vi "GPIB Send Receive.vi"(1 "RDY max wait, ms":u32=500, 4 "RDY when up":bool=TRUE, 5 "Data ready bit (-1 - ignore)":i32=-1, 6 "Read terminator":i16, 7 "Delay, ms":u32, 8 "error in (no error)":errorcluster, 9 "Receive count":i32=256, 10 "data string in":string, 11 "GPIB Adress":i16) -> (0 "error out":errorcluster, 2 "data string out":string, 3 "GPIB Adress out":i16)   [LabVIEW 2019]
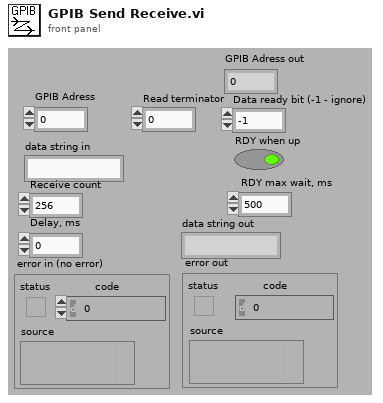
[diagram p1: front panel]
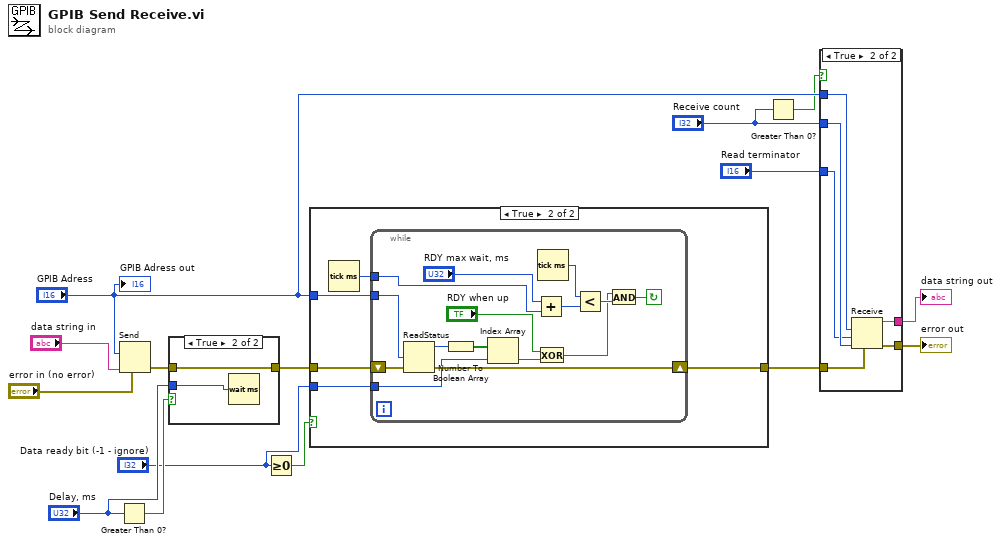
[diagram p0: block diagram]
diagram:
  n1 = Greater Than 0?(x="Delay, ms") -> (x > 0?=w11:bool)
  n2 = Send(2:"GPIB Adress", 4:"error in (no error)", 5:"data string in") -> (8:w10:errorcluster)  [unwired: 4 out]
  n3 = case shown="True" w11 {
    tunnel: w10 -> [w16 w17]
    tunnel: [w16 w17] -> w5
    tunnel: "Delay, ms" -> [_ w18]
    frame False {
    }
    frame True {
      n4 = Wait (ms)(milliseconds to wait=w18) -> ()  [unwired: 1 out]
    }
  }
  n5 = Greater Or Equal To 0?(x="Data ready bit (-1 - ignore)") -> (x >= 0?=w7:bool)
  n6 = case shown="True" w7 {
    tunnel: "GPIB Adress" -> [_ w23]
    tunnel: w5 -> [w19 w22]
    tunnel: "Data ready bit (-1 - ignore)" -> [_ w21]
    tunnel: [w19 w20] -> w3
    frame False {
    }
    frame True {
      n7 = Tick Count (ms)() -> (millisecond timer value=w24:u32)
      n8 = while {
        tunnel: w23 -> [w38]
        shift-right: [w37] -> w20
        shift-left: w22 -> [w39]
        tunnel: w24 -> [w32]
        tunnel: w21 -> [w28]
        stop <- w36 continue-if-true
        n9 = ReadStatus(3:w39, 4:w38) -> (0:w37:errorcluster, 2:w34:i16)  [unwired: 2 out]
        n10 = Number To Boolean Array(number=w34) -> (Boolean array=w30:bool[])
        n11 = Index Array(array=w30, index=w28) -> (element=w27:bool)
        n12 = Add(x="RDY max wait, ms", y=w32) -> (x+y=w33:u32)
        n13 = Exclusive Or(1:w27, 2:"RDY when up") -> (0:w26:bool)
        n14 = Tick Count (ms)() -> (millisecond timer value=w31:u32)
        n15 = Less?(x=w31, y=w33) -> (x < y?=w35:bool)
        n16 = And(x=w26, y=w35) -> (x .and. y?=w36:bool)
      }
    }
  }
  n17 = Greater Than 0?(x="Receive count") -> (x > 0?=w1:bool)
  n18 = case shown="True" w1 {
    tunnel: [w40 w46] -> w14
    tunnel: [_ w45] -> w13
    tunnel: "Receive count" -> [_ w44]
    tunnel: "Read terminator" -> [_ w43]
    tunnel: "GPIB Adress" -> [_ w42]
    tunnel: w3 -> [w40 w41]
    frame False {
    }
    frame True {
      n19 = Receive(4:w41, 6:w44, 7:w43, 8:w42) -> (0:w46:errorcluster, 3:w45:string)  [unwired: 3 out]
    }
  }
  "error out" <- w14
  "data string out" <- w13
  "GPIB Adress out" <- "GPIB Adress"
